vi "Write Measurements Menu.vi"(8 "error in (no error)":errorcluster, 10 "Measurements Menu":refnum<vi>, 11 "Common Measurements Interface in":refnum<class "Common Measurements Interface.lvclass">) -> (0 "error out":errorcluster, 3 "Common Measurements Interface out":refnum<class "Common Measurements Interface.lvclass">)   [LabVIEW 2015, in "Common Measurements Interface.lvclass"]
uses:
  Common Measurements Interface.lvclass
  Queued Listbox/Queued Listbox.xctl
  Common Measurements Interface.lvclass/Common Measurements Interface.ctl
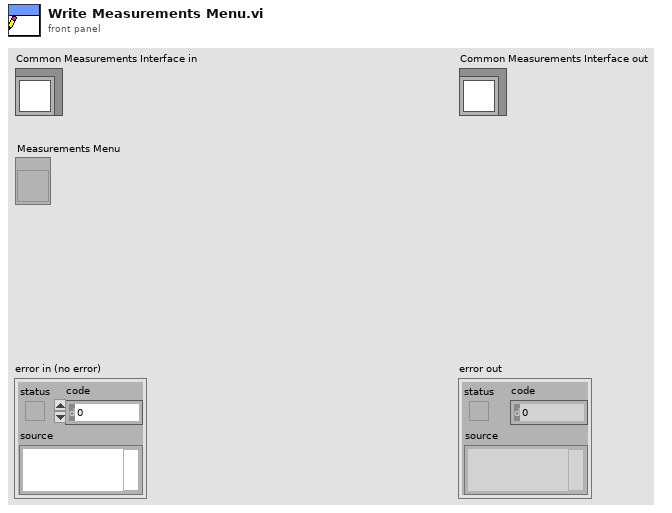
[diagram p1: front panel]
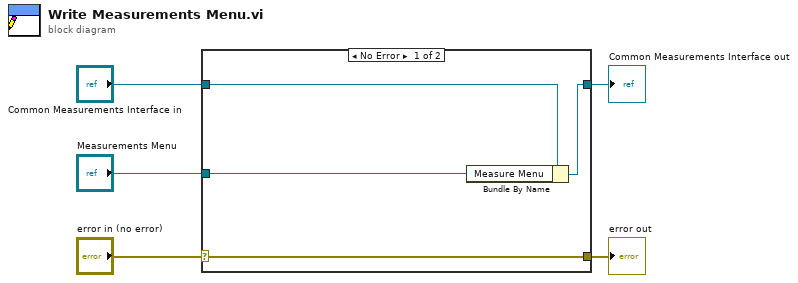
[diagram p0: block diagram]
diagram:
  n1 = case shown="No Error" "error in (no error)" {
    selector: "error in (no error)" -> [w9 w10]
    tunnel: [w9 w10] -> w4
    tunnel: [w7 w11] -> w2
    tunnel: "Common Measurements Interface in" -> [w8 w11]
    tunnel: "Measurements Menu" -> [w6 _]
    frame No Error {
      n2 = Bundle By Name(cluster=w8, "Measure Menu"=w6) -> (w7:refnum<class "Common Measurements Interface.lvclass">)
    }
    frame Error {
    }
  }
  "error out" <- w4
  "Common Measurements Interface out" <- w2
